vi "SaveCallibrationResults.vi"(9 "Peak (left)":dbl, 10 "Peak (right)":dbl, 11 "Peak position":dbl) -> ()   [LabVIEW 2013]
uses:
  <vilib>/Utility/file.llb/Write To Spreadsheet File (DBL).vi
panel:
  out "Application Directory":path
  out "appended array":dbl[](array[numeric])
  out "appended path":path
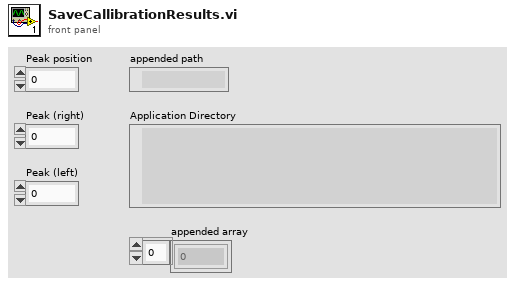
[diagram p1: front panel]
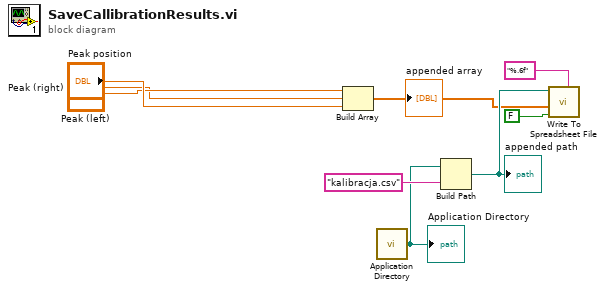
[diagram p0: block diagram]
diagram:
  n1 = Build Array("Peak (left)", "Peak (right)", "Peak position") -> (w4:dbl[])
  "appended array" <- w4
  n2 = call <vilib>:"Application Directory.vi"() -> ("Application Directory"=w7:path)
  "Application Directory" <- w7
  n3 = Build Path(base path=w7, name or relative path="kalibracja.csv") -> (appended path=w9:path)
  "appended path" <- w9
  n4 = call-poly <vilib>:"Write To Spreadsheet File.vi"("format (%.3f)"="%.6f", "append to file? (new file:F)"=FALSE, "1D data"=w4, "file path (dialog if empty)"=w9) -> ()  [unwired: 4 in, 1 out]
